vi "ManualL1Control_IPR.vi"() -> ()   [LabVIEW 2012]
uses:
  <vilib>/Utility/NIReport.llb/NI_report.lvclass
  <vilib>/Utility/NIReport.llb/HTML/NI_HTML.lvclass
panel:
  out "IPR_count":u32
  in  "DAC_TH1":u32(slide)=255 max=255 step=1 scale=0.0..255.0
  in  "DAC_TH0":u32(slide)=255 max=255 step=1 scale=0.0..255.0
  in  "DAC_TH2":u32(slide)=255 max=255 step=1 scale=0.0..255.0
  in  "stop":bool
  in  "Instrument VISA in":T1={"AWG VISA"="AgilentGenerator1", "Oscilloscope  VISA "="AgilentOsciloscope", "Integration Board IP"="172.16.17.48", "connection ID"=refnum, "report out"=refnum, "report file path"=path "C:/Documents and Settings/CTA_LAB01/Desktop/L0_Asic/L0 Asic Test Data"}
  in  "SingleIN/#Combination":bool=TRUE
  in  "Combination":i32 min=0 max=127 step=1 format="%b"
  in  "! All Channels (false activates all channels)":bool=TRUE
  in  "Enable  L1 single  Input":i32(slide) scale=0.0..6.0
  in  "error in":errorcluster
  out "data out serial":string="writtingwritting2"
  out "error out":errorcluster
  out "REG Array":u32[](array[numeric])=[6826, 65535, 65535, 65535, 65023, 383, 13312]
  in  "Register Adress 96":bool[](array[boolean])=[FALSE, TRUE, FALSE, TRUE, FALSE, TRUE, FALSE, TRUE, FALSE, TRUE, FALSE, TRUE, TRUE, FALSE, FALSE, FALSE]
  out "REG 96":u32=6826
  out "?":bool[](array[boolean])=[TRUE, TRUE, TRUE, TRUE, TRUE, TRUE, TRUE, TRUE, TRUE, TRUE, TRUE, TRUE, TRUE, TRUE, TRUE, TRUE, FALSE, FALSE, FALSE, FALSE, FALSE, FALSE, FALSE, FALSE, FALSE, FALSE, FALSE, FALSE, FALSE, FALSE, FALSE, FALSE, FALSE, FALSE, FALSE, FALSE, FALSE, FALSE, FALSE, FALSE, FALSE, FALSE, FALSE, FALSE, FALSE, FALSE, FALSE, FALSE, FALSE, FALSE, FALSE, FALSE, FALSE, FALSE, FALSE, FALSE, FALSE, FALSE, FALSE, FALSE, FALSE, FALSE, FALSE, FALSE]
  out "REG 99":u32=65535
  in  "DAC_TH4":u32=255
  out "?":bool[](array[boolean])=[TRUE, TRUE, TRUE, TRUE, TRUE, TRUE, TRUE, TRUE, TRUE, TRUE, TRUE, TRUE, TRUE, TRUE, TRUE, TRUE, FALSE, FALSE, FALSE, FALSE, FALSE, FALSE, FALSE, FALSE, FALSE, FALSE, FALSE, FALSE, FALSE, FALSE, FALSE, FALSE, FALSE, FALSE, FALSE, FALSE, FALSE, FALSE, FALSE, FALSE, FALSE, FALSE, FALSE, FALSE, FALSE, FALSE, FALSE, FALSE, FALSE, FALSE, FALSE, FALSE, FALSE, FALSE, FALSE, FALSE, FALSE, FALSE, FALSE, FALSE, FALSE, FALSE, FALSE, FALSE]
  out "REG 98":u32=65535
  in  "DAC_TH3":u32=255
  out "?":bool[](array[boolean])=[TRUE, TRUE, TRUE, TRUE, TRUE, TRUE, TRUE, TRUE, TRUE, TRUE, TRUE, TRUE, TRUE, TRUE, TRUE, TRUE, FALSE, FALSE, FALSE, FALSE, FALSE, FALSE, FALSE, FALSE, FALSE, FALSE, FALSE, FALSE, FALSE, FALSE, FALSE, FALSE, FALSE, FALSE, FALSE, FALSE, FALSE, FALSE, FALSE, FALSE, FALSE, FALSE, FALSE, FALSE, FALSE, FALSE, FALSE, FALSE, FALSE, FALSE, FALSE, FALSE, FALSE, FALSE, FALSE, FALSE, FALSE, FALSE, FALSE, FALSE, FALSE, FALSE, FALSE, FALSE]
  out "REG 97":u32=65535
  in  "DAC_TH5":u32=255
  in  "Register Adress 102":bool[](array[boolean])=[FALSE, FALSE, FALSE, FALSE, FALSE, FALSE, FALSE, FALSE, FALSE, FALSE, TRUE, FALSE, TRUE, TRUE, FALSE, FALSE]
  out "REG 102":u32=13312
  in  "Register Adress 101":bool[](array[boolean])=[TRUE, TRUE, TRUE, TRUE, TRUE, TRUE, TRUE, FALSE, TRUE, FALSE, FALSE, FALSE, FALSE, FALSE, FALSE, FALSE]
  out "REG 101":u32=383
  in  "Register Adress 100":bool[](array[boolean])=[TRUE, TRUE, TRUE, TRUE, TRUE, TRUE, TRUE, TRUE, TRUE, FALSE, TRUE, TRUE, TRUE, TRUE, TRUE, TRUE]
  out "REG 100":u32=65023
  # "0           1            2"
  # "DAC_TH0"
  # "DAC_TH1"
  # "DAC_TH2"
  # "DAC_TH3"
  # "DAC_TH4"
  # "DAC_TH5"
  # "Unused"
  # "DAC_MUX_ENA"
  # "ADDER_C"
  # "ADDER_A"
  # "ADDER_B"
  # "a         b         c"
  # "a         b         c"
  # "a         b         c"
  # "a         b         c"
  # "a         b         c"
  # "Unused"
  # "CH0"
  # "CH1"
  # "CH2"
  # "CH3"
  # "CH4"
  # "a         b         c"
  # "ENA_0  ENA_1"
  # "ENA_0  ENA_1"
  # "a         b         c"
  # "BUFF\nENA"
  # "R       E       S      E        R     V        E      D"
  # "MUX"
  # "LVDS"
  # "CH5"
  # "CH6"
  # "R               E               S               E                  R                V             E              D"
  # "0            1            2            3           4             5"
  # "DAC _IB"
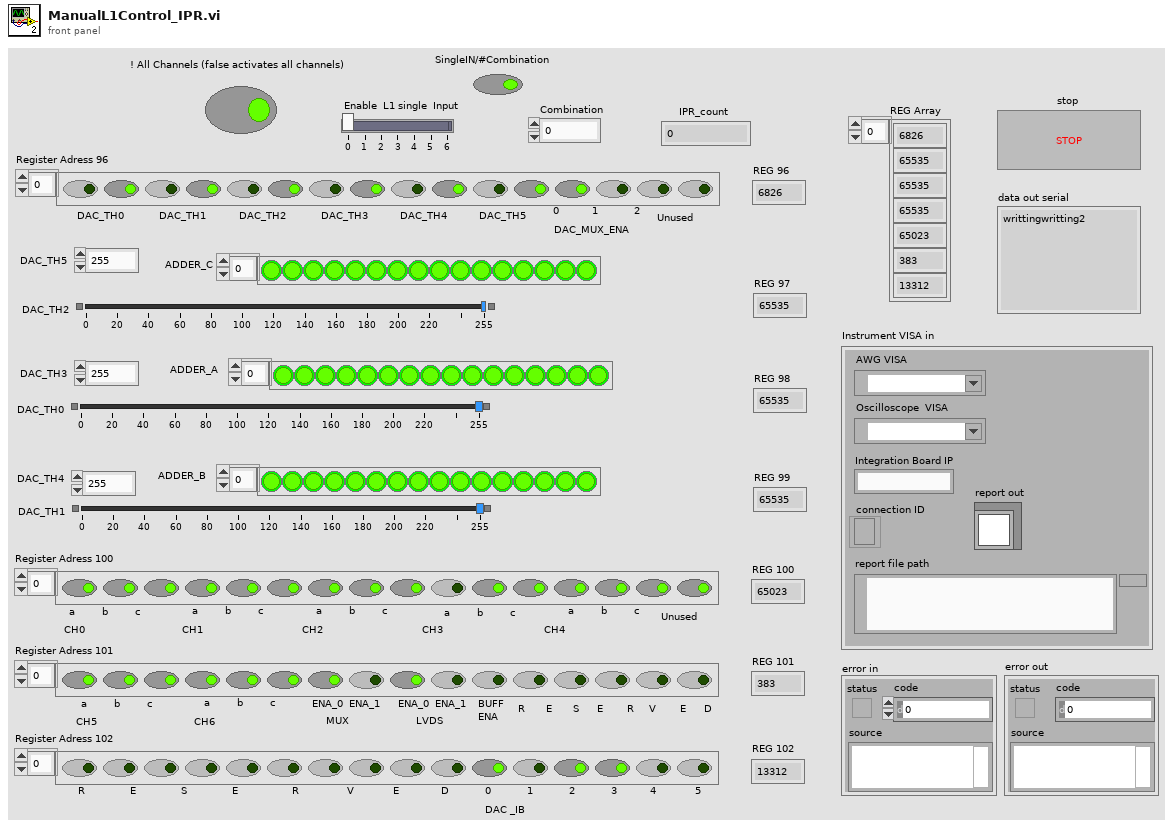
[diagram p1: front panel]
types:
  T1 = cluster{"AWG VISA":refnum<visa-resource-name>, "Oscilloscope  VISA ":refnum<visa-resource-name>, "Integration Board IP":string, "connection ID":refnum<k5>, "report out":refnum<class "NI_report.lvclass">, "report file path":path}
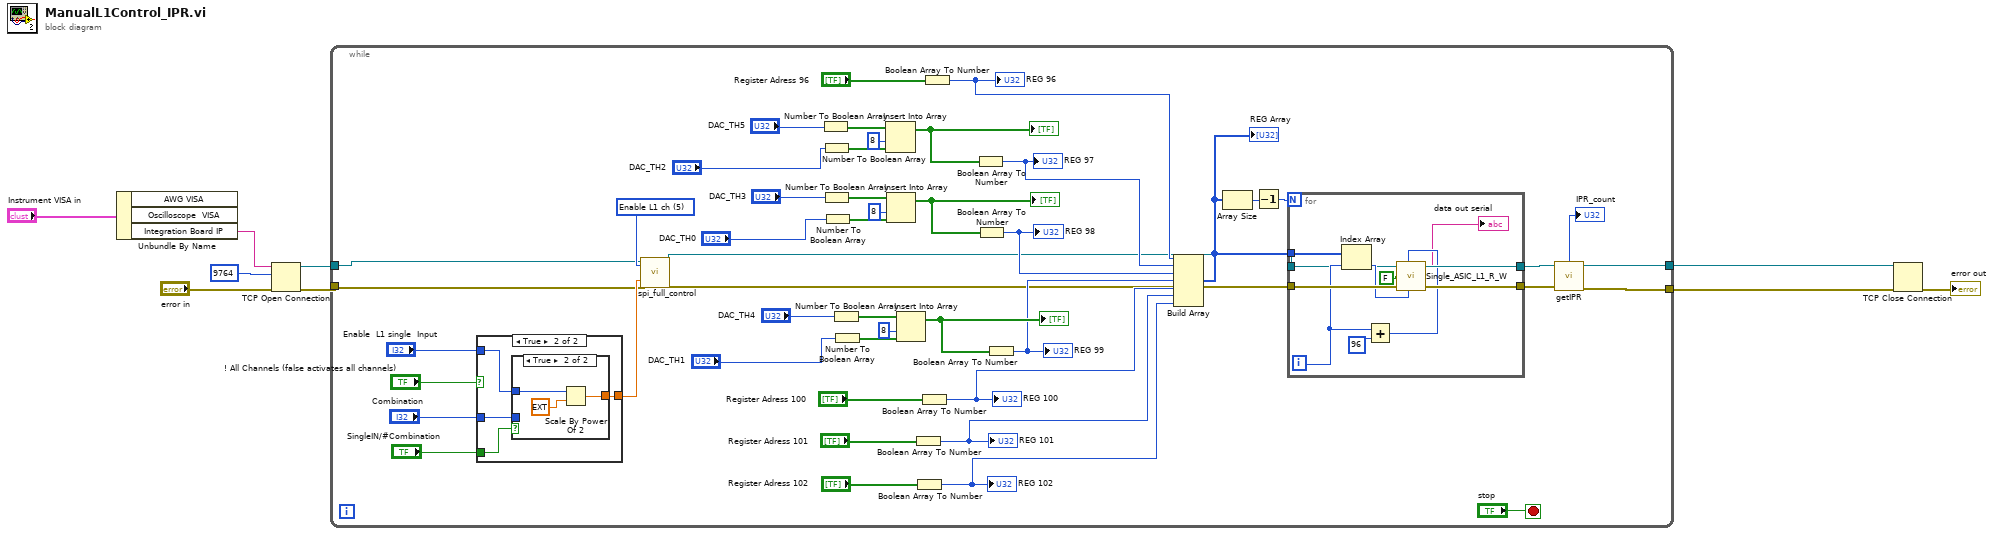
[diagram p0: block diagram]
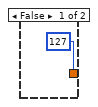
[diagram p2: hidden frame]
diagram:
  n1 = Unbundle By Name("Instrument VISA in") -> ("Integration Board IP"=w8:string)  [unwired: 2 out]
  n2 = TCP Open Connection(address=w8, remote port or service name=9764, error in (no error)="error in") -> (connection ID=w4:refnum<k5>, error out=w2:errorcluster)  [unwired: 2 in]
  n3 = while {
    tunnel: w2 -> [w21]
    tunnel: [w12] -> w3
    tunnel: w4 -> [w22]
    tunnel: [w10] -> w1
    stop <- "stop" stop-if-true
    w28 = u16 5 items=["Attenuation", "Clipping", "Enable channel", "Delay line", "ASIC", "Enable L1 ch", "ASIC L1"] ("Device")
    n4 = case shown="True" "! All Channels (false activates all channels)" {
      tunnel: [127 ("Register or channel") w61] -> w29
      tunnel: "Enable  L1 single  Input" -> [_ w62]
      tunnel: "Combination" -> [_ w60]
      tunnel: "SingleIN/#Combination" -> [_ w59]
      frame False {
      }
      frame True {
        n5 = case shown="True" w59 {
          tunnel: w62 -> [_ w65]
          tunnel: [w63 w64] -> w61
          tunnel: w60 -> [w63 _]
          frame False {
          }
          frame True {
            n6 = Scale By Power Of 2(n=w65, x=ext 1.0) -> (x*2^n=w64:ext)
          }
        }
      }
    }
    n7 = call "spi_full_control.vi"("connection ID"=w22, "Device"=w28, "Data"=w29, "error out 3"=w21) -> ("connection ID out"=w23:refnum<k5>, "error out 2"=w24:errorcluster)  [unwired: 8 in, 6 out]
    n8 = Number To Boolean Array(number="DAC_TH5") -> (Boolean array=w53:bool[])
    n9 = Number To Boolean Array(number="DAC_TH2") -> (Boolean array=w52:bool[])
    n10 = Number To Boolean Array(number="DAC_TH3") -> (Boolean array=w48:bool[])
    n11 = Number To Boolean Array(number="DAC_TH0") -> (Boolean array=w47:bool[])
    n12 = Number To Boolean Array(number="DAC_TH4") -> (Boolean array=w43:bool[])
    n13 = Number To Boolean Array(number="DAC_TH1") -> (Boolean array=w42:bool[])
    n14 = Insert Into Array(array=w53, index=8, new element=w52) -> (w51:bool[])
    "?" <- w51
    n15 = Insert Into Array(array=w48, index=8, new element=w47) -> (w46:bool[])
    "?" <- w46
    n16 = Insert Into Array(array=w43, index=8, new element=w42) -> (w41:bool[])
    "?" <- w41
    n17 = Boolean Array To Number(Boolean array="Register Adress 101") -> (number=w33:u32)
    "REG 101" <- w33
    n18 = Boolean Array To Number(Boolean array="Register Adress 102") -> (number=w32:u32)
    "REG 102" <- w32
    n19 = Boolean Array To Number(Boolean array="Register Adress 100") -> (number=w34:u32)
    "REG 100" <- w34
    n20 = Boolean Array To Number(Boolean array="Register Adress 96") -> (number=w38:u32)
    "REG 96" <- w38
    n21 = Boolean Array To Number(Boolean array=w51) -> (number=w37:u32)
    "REG 97" <- w37
    n22 = Boolean Array To Number(Boolean array=w46) -> (number=w36:u32)
    "REG 98" <- w36
    n23 = Boolean Array To Number(Boolean array=w41) -> (number=w35:u32)
    "REG 99" <- w35
    n24 = Build Array(w38, w37, w36, w35, w34, w33, w32) -> (w31:u32[])
    "REG Array" <- w31
    n25 = Array Size(array=w31) -> (size(s)=w16:i32)
    n26 = Decrement(x=w16) -> (x-1=w15:i32)
    n27 = for {
      N: w15 -> [_]
      tunnel: w24 -> [w77]
      tunnel: w31 -> [w76]
      tunnel: [w75] -> w11
      tunnel: [w74] -> w13
      tunnel: w23 -> [w67]
      i -> [w70]
      n28 = Index Array(array=w76, index=w70) -> (element=w73:u32)
      n29 = Add(x=w70, y=96) -> (x+y=w71:i32)
      n30 = call "Single_ASIC_L1_R_W.vi"("connection ID"=w67, "Register or channel"=w71, "RD/#WR"=FALSE, "error in (no error)"=w77, "Data"=w73) -> ("data out serial"=→"data out serial":string, "connection ID out"=w75:refnum<k5>, "error out"=w74:errorcluster)  [unwired: 1 in, 1 out]
    }
    n31 = call "getIPR.vi"("error in"=w13, "connection ID"=w11) -> ("error out"=w12:errorcluster, "connection ID out"=w10:refnum<k5>, "IPR_count"=→"IPR_count":u32)  [unwired: 6 in, 1 out]
  }
  n32 = TCP Close Connection(connection ID=w1, error in (no error)=w3) -> (error out=→"error out":errorcluster)  [unwired: 1 in, 1 out]
